vi "Init.vi"(8 "error in":errorcluster, 11 "object in":refnum<class "SDS1022 Base CFG.lvclass">) -> (0 "error out":errorcluster, 3 "object out":refnum<class "SDS1022 Base CFG.lvclass">)   [LabVIEW 2023, in "OWON SDS1022.lvlib" / "SDS1022 Base CFG.lvclass"]
uses:
  SDS1022 Base CFG.lvclass
  D:/git/HAL/Scope VISA/Configuration/Scope VISA CFG.lvclass
  HAL/Scope VISA/Configuration/Scope VISA CFG.lvclass/Scope VISA CFG.ctl
  HAL/Scope VISA/Configuration/Scope VISA CFG.lvclass
  SDS1022 Base CFG.lvclass/SDS1022 Base CFG.ctl
  D:/git/HAL/Configuration Base/Configuration Base.lvclass
  D:/git/HAL/Interfaces/IConfigure/IConfigure.lvclass
  D:/git/HAL/Interfaces/IConfigure Scope/IConfigure Scope.lvclass
  D:/git/OWON-SDS1022-LabVIEW/OWON SDS1022/Configurations/SDS1000 Base CFG/SDS1022 Base CFG.lvclass
panel:
  out "Instrument ID":string
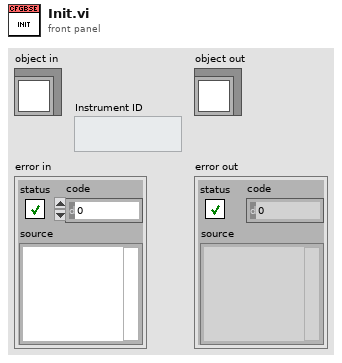
[diagram p1: front panel]
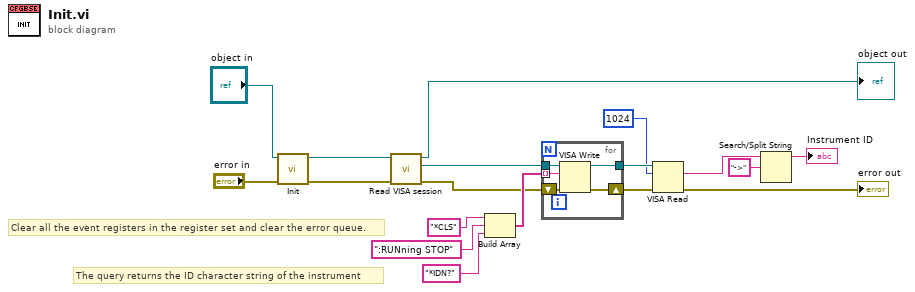
[diagram p0: block diagram]
diagram:
  # "The query returns the ID character string of the instrument"
  # "Clear all the event registers in the register set and clear the error queue."
  n1 = call-parent "Init.vi"("error in"="error in", "Scope VISA CFG in"="object in") -> ("error out"=w2:errorcluster, "Scope VISA CFG out"=w1:refnum<class "SDS1022 Base CFG.lvclass">)  [unwired: 8 in]
  n2 = call "Read VISA session.vi"("error in (no error)"=w2, "Scope VISA CFG in"=w1) -> ("error out"=w3:errorcluster, "VISA session"=w4:refnum<visa-resource-name>, "Scope VISA CFG out"=→"object out":refnum<class "SDS1022 Base CFG.lvclass">)  [unwired: 7 in]
  n3 = Build Array("*CLS" ("write buffer"), ":RUNning STOP" ("element"), "*IDN?") -> (w15:string[])
  n4 = for {
    tunnel: w15 -> [w22] mode=indexing
    shift-right: [w21] -> w12
    shift-left: w3 -> [w23]
    tunnel: [w20] -> w7
    tunnel: w4 -> [w19]
    n5 = VISA Write(VISA resource name=w19, write buffer=w22, error in (no error)=w23) -> (VISA resource name out=w20:refnum<visa-resource-name>, error out=w21:errorcluster)  [unwired: 1 out]
  }
  n6 = VISA Read(VISA resource name=w7, byte count=u32 1024, error in (no error)=w12) -> (read buffer=w10:string, error out=→"error out":errorcluster)  [unwired: 2 out]
  n7 = Search/Split String(string=w10, search string/char (-)="->") -> (substring before match=→"Instrument ID":string)  [unwired: 1 in, 2 out]
